vi "John Shutter Control.vi"(2 "input error":errorcluster, 3 "Shutter":bool) -> (0 "error out":errorcluster)   [LabVIEW 2009]
panel:
  out "Ready to go":bool
  in  "Set":bool
  in  "stop":bool
  # "Takes about 20-25 seconds to start..wait until \"Ready to go\" turns green..."
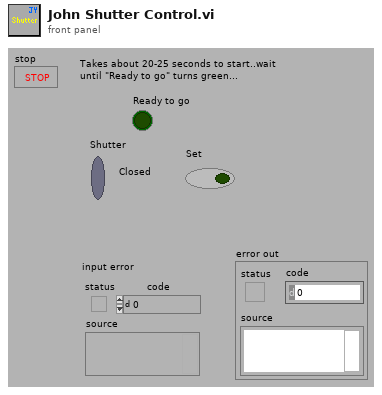
[diagram p1: front panel]
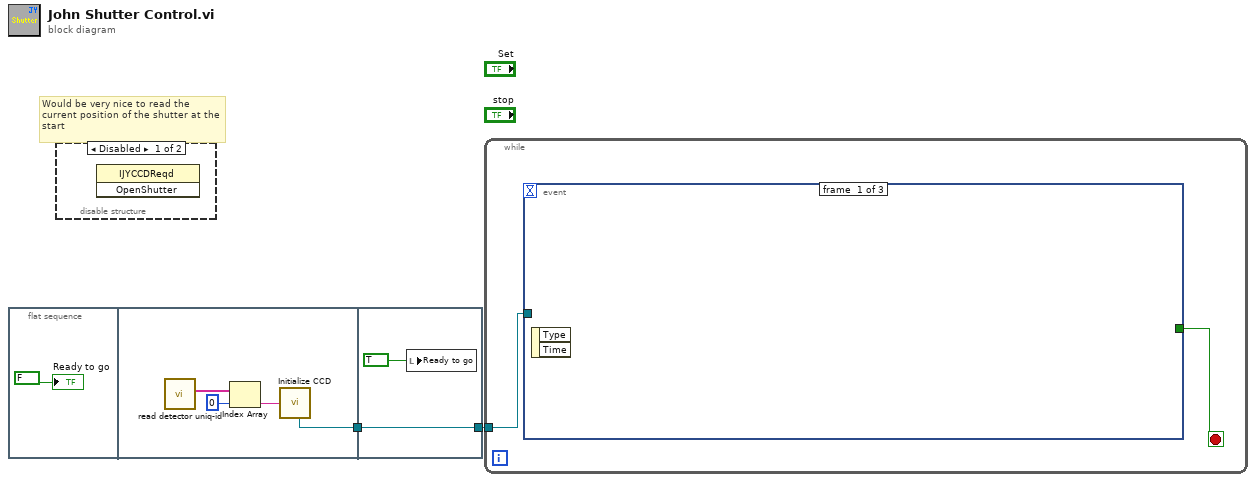
[diagram p0: block diagram]
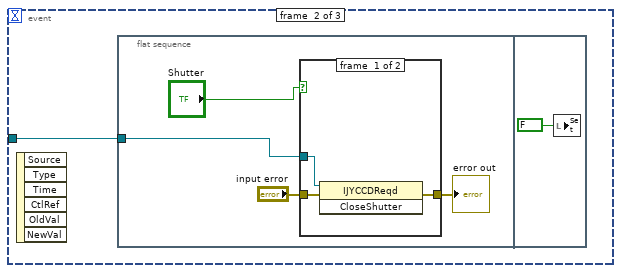
[diagram p3: hidden frame]
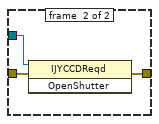
[diagram p4: hidden frame]
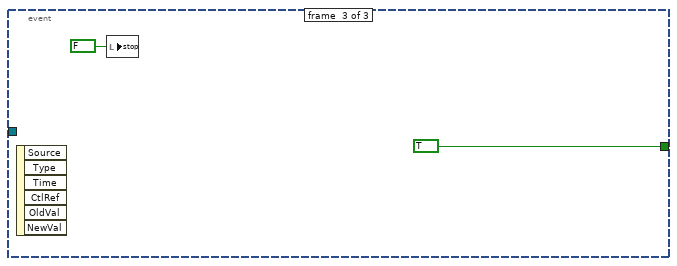
[diagram p5: hidden frame]
diagram:
  # "Would be very nice to read the current position of the shutter at the start"
  n1 = flat-sequence {
    tunnel: [w4] -> w1
    tunnel: [w9] -> w2
    tunnel: w1 -> [w9]
    frame #0 {
      "Ready to go" <- FALSE
    }
    frame #1 {
      n2 = call "read detector uniq-id.vi"() -> ("UniqueID"=w5:string[])  [unwired: 6 out]
      n3 = Index Array(array=w5, index=0) -> (element=w7:string)
      n4 = call "Initialize CCD.vi"("Unique id:"=w7) -> ("JYCCDLib.IJYCCDReqd"=w4:refnum<k7>)  [unwired: 7 out]
    }
    frame #2 {
      n5 = local write "Ready to go"(TRUE) -> ()
    }
  }
  n6 = disable-structure shown="Disabled" {
    frame #0 {
      n7 = invoke class="IJYCCDReqd" method="OpenShutter"() -> ()  [unwired: 3 in, 3 out]
    }
    frame #1 {
    }
  }
  n8 = while {
    tunnel: w2 -> [w10]
    stop <- w11 stop-if-true
    n9 = event shown="[1] \"Set\": Value Change" {
      selector: _ -> [_ _ _]
      dyn-events: _ -> [_ _ _]
      timeout: _ -> [_ _ _]
      tunnel: [_ _ TRUE] -> w11
      tunnel: w10 -> [_ w12 _]
      event #0 {
        n10 = event-data() -> ()  [unwired: 3 out]
      }
      event #1 {
        n11 = event-data() -> ()  [unwired: 7 out]
        n12 = flat-sequence {
          tunnel: w12 -> [w14]
          frame #0 {
            n13 = case shown="False" "Shutter" {
              tunnel: [w19 w22] -> w16
              tunnel: "input error" -> [w18 w21]
              tunnel: w14 -> [w17 w20]
              frame #0 {
                n14 = invoke class="IJYCCDReqd" method="CloseShutter"(reference=w17, error in=w18) -> (error out=w19:errorcluster)  [unwired: 1 in, 2 out]
              }
              frame #1 {
                n15 = invoke class="IJYCCDReqd" method="OpenShutter"(reference=w20, error in=w21) -> (error out=w22:errorcluster)  [unwired: 1 in, 2 out]
              }
            }
            "error out" <- w16
          }
          frame #1 {
            n16 = local write "Set"(FALSE) -> ()
          }
        }
      }
      event #2 {
        n17 = event-data() -> ()  [unwired: 7 out]
        n18 = local write "stop"(FALSE) -> ()
      }
    }
  }
